vi "CVSUI.vi"() -> ()   [LabVIEW 2013, in "PLTarget CVS.lvclass"]
uses:
  PLTarget CVS.lvclass
  <vilib>/NI/Configuration Framework/Node/NodeRef.ctl
  <vilib>/NI/Configuration Framework/Node/NISE_CEF_Node.lvclass
  <vilib>/NI/AMC/Message Queue.ctl
  <vilib>/NI/AMC/Message.ctl
  <vilib>/NI/Tools/Keyed Array/KeyedArray.ctl
  <vilib>/NI/Configuration Framework/Node/UserEventRef.ctl
  <vilib>/NI/Configuration Framework/Controls/EventCluster.ctl
  <vilib>/NI/Tag Bus Module Framework/root configuration/Target Types.ctl
  <vilib>/NI/Configuration Framework/Node/RefreshUIEvent.ctl
  <vilib>/NI/Configuration Framework/Node/CacheState.ctl
  <vilib>/NI/Configuration Framework/Node/StopEvent.ctl
  <vilib>/NI/Configuration Framework/Node/NodeChangeEvent.ctl
  Configuration Editor/Classes/TBM Configuration Node/deployment configuration.ctl
  Configuration Editor/Classes/Targets/Targets.lvclass/Targets.ctl
  PLTarget CVS.lvclass/PLTarget CVS.ctl
  Framework Configuration Classes/target configuration/PL_Target Configuration.lvclass/PL_Target Configuration.ctl
  <vilib>/NI/Configuration Framework/serializable node/NISE_CEF_serializable node.lvclass
  <vilib>/NI/Tag Bus Module Framework/root configuration/TBM configuration.lvclass
  Configuration Editor/Classes/Targets/Write additional files.vi
  Configuration Editor/Classes/Targets/Read additional files.vi
  <vilib>/NI/Configuration Framework/serializable configuration/set alias.vi
  <vilib>/NI/Configuration Framework/serializable configuration/get alias.vi
  <vilib>/NI/Configuration Framework/serializable configuration/NISE_CEF_serializable configuration.lvclass
  Framework Configuration Classes/target configuration/PL_Target Configuration.lvclass
  Configuration Editor/Classes/Targets/Targets.lvclass
  <vilib>/NI/Tools/Keyed Array/Tools_KeyedArray.lvlib
  <vilib>/NI/AMC/AMC.lvlib
  <vilib>/NI/Configuration Framework/NISE_CEF_TreeControl.lvlib
  Configuration Editor/Classes/TBM Configuration Node/TBM Configuration Node.lvclass
panel:
  in  "additional files":T1[](array[typedef])
  in  "node change":T2
  in  "stop event":T3
  in  "cache state":T4
  in  "refresh UI":T5
  in  "open fp?":bool=TRUE
  in  "generate includes file":bool
  in  "Includes file path":path
  in  "Local Bitfile Path":path
  in  "load bitfile":bool
  in  "bitfile path on target relative to root (c:\\ or /home/lvuser/)":path
  in  "RIO FPGA":string="RIO0"
  in  "Target Type":T6=enum."Linux RT ARM"
  in  "path to deploy on target relative to root (c:\\ or /home/lvuser/)":path
  in  "IP":string
  in  "user event":T7
  in  "main queue":T8
  in  "Name":string
  in  "node ref":T9
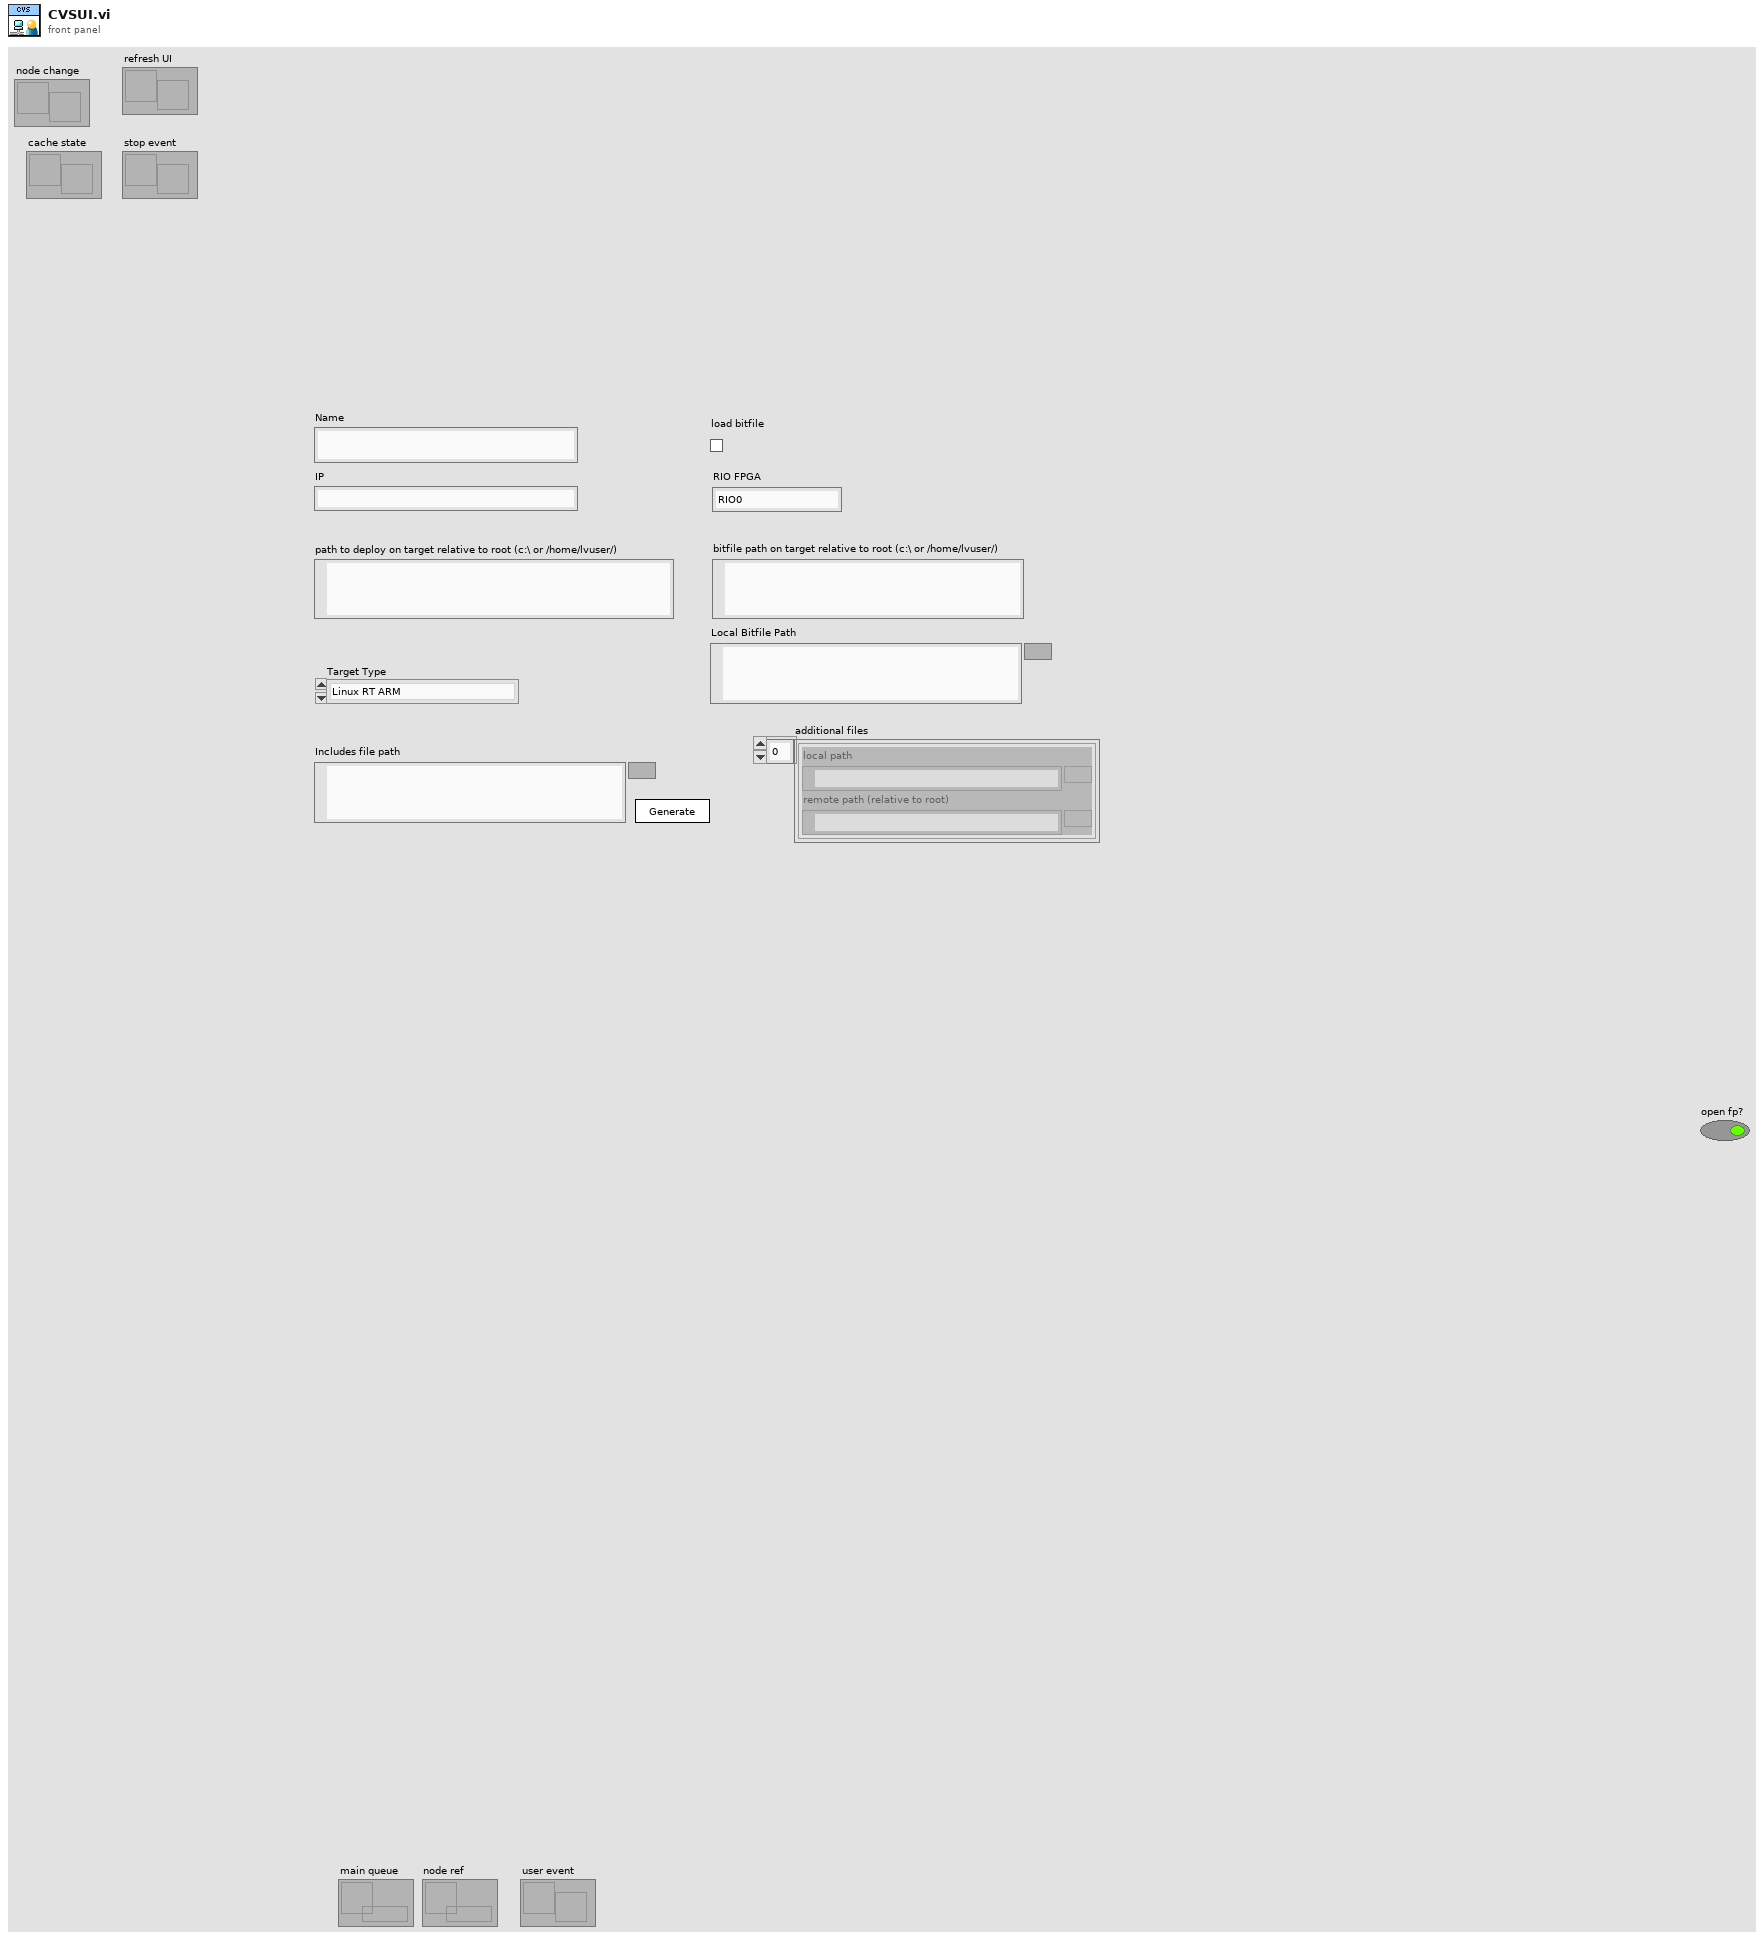
[diagram p1: front panel]
types:
  T1 = typedef "PL Framework Configuration Tool.lvlib/TBM Configuration Node.lvclass/deployment configuration.ctl" = cluster{"local path":path, "remote path (relative to root)":path}
  T2 = typedef "NISE_CEF_Node.lvclass/NodeChangeEvent.ctl" = refnum<user-event>
  T3 = typedef "NISE_CEF_Node.lvclass/StopEvent.ctl" = refnum<user-event>
  T4 = typedef "NISE_CEF_Node.lvclass/CacheState.ctl" = refnum<user-event>
  T5 = typedef "NISE_CEF_Node.lvclass/RefreshUIEvent.ctl" = refnum<user-event>
  T6 = typedef "TBM configuration.lvclass/Target Types.ctl" = enum16{"Windows", "Mac", "Linux", "Linux RT ARM", "VxWorks", "Pharlap", "Other", "Linux RT x64"}
  T7 = typedef "NISE_CEF_Node.lvclass/UserEventRef.ctl" = refnum<user-event>
  T8 = typedef "AMC.lvlib/Message Queue.ctl" = refnum<queue>
  T9 = typedef "NISE_CEF_Node.lvclass/NodeRef.ctl" = refnum<data-value>
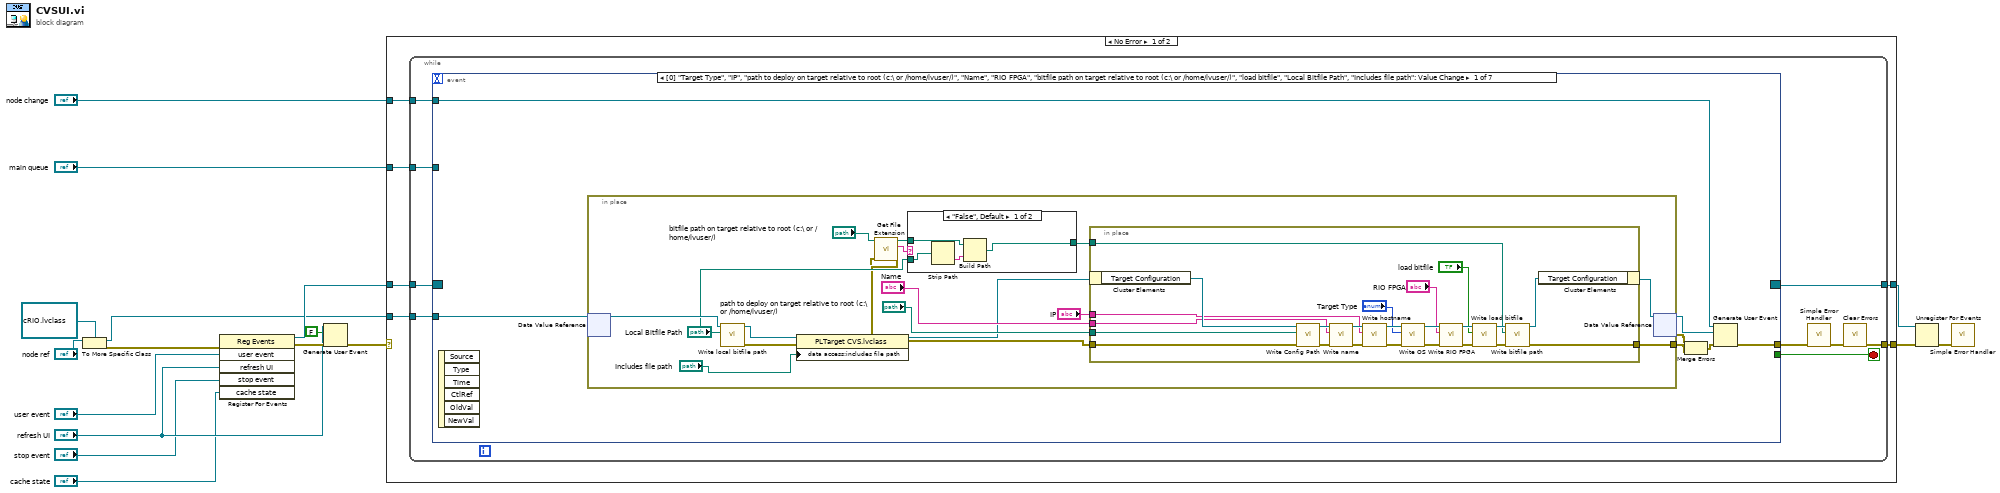
[diagram p0: block diagram]
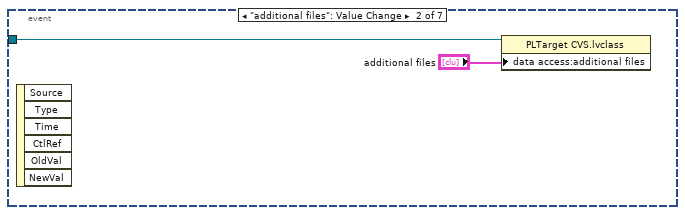
[diagram p3: hidden frame]
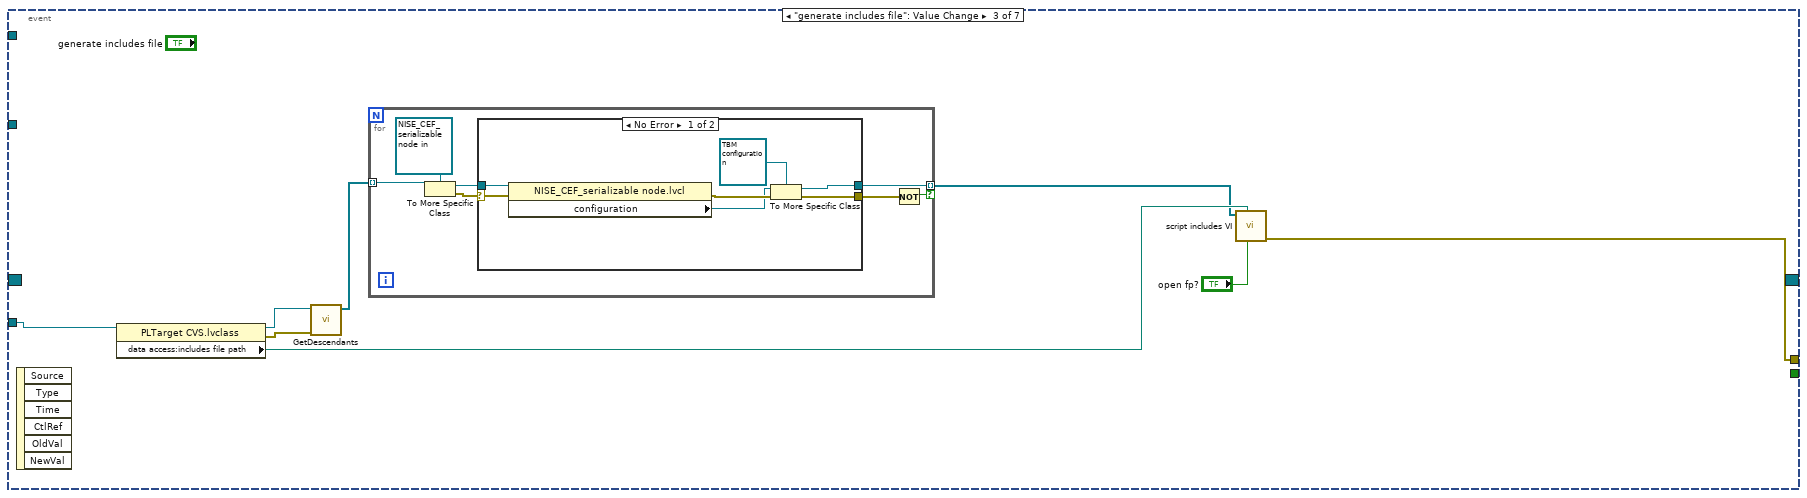
[diagram p4: hidden frame]
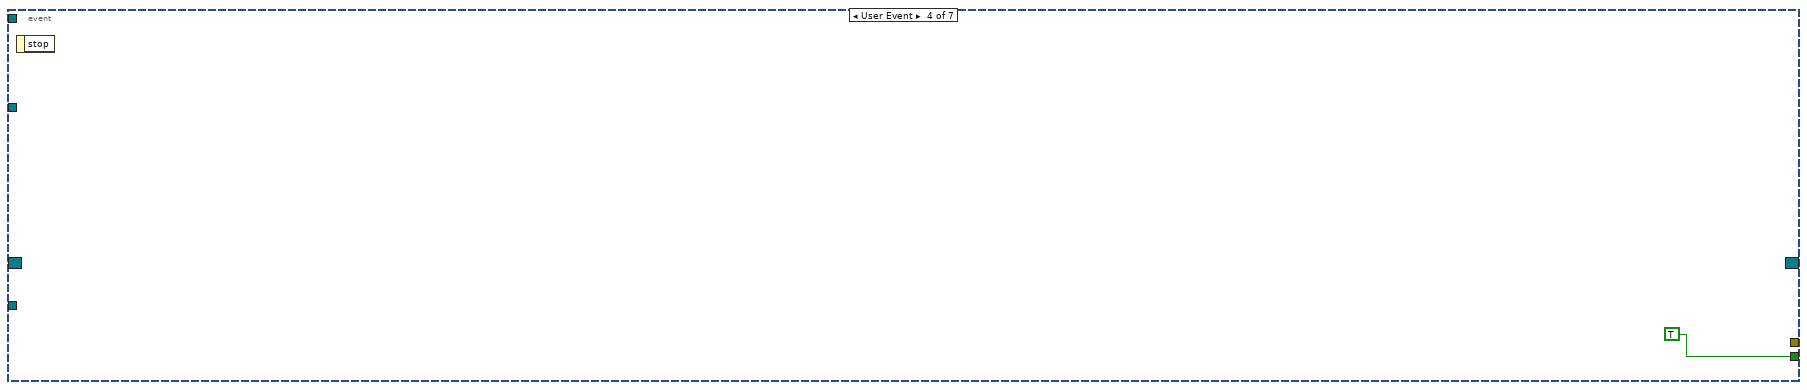
[diagram p6: hidden frame]
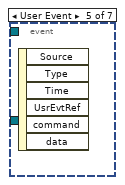
[diagram p7: hidden frame]
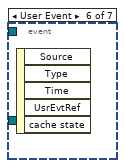
[diagram p8: hidden frame]
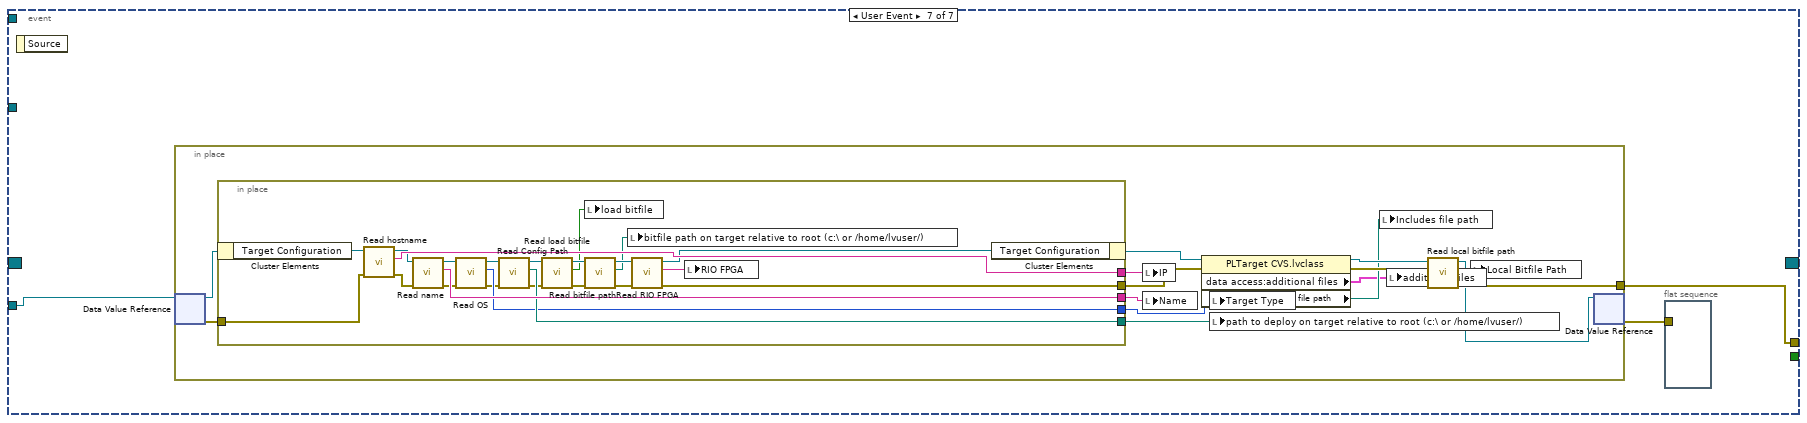
[diagram p9: hidden frame]
diagram:
  n1 = To More Specific Class(target class=refnum<data-value> refnum ("data value reference"), reference="node ref") -> (specific class reference=w4:refnum<data-value>, error out=w5:errorcluster)  [unwired: 1 in]
  n2 = register-events(error in=w5, "user event", "refresh UI", "stop event", "cache state") -> (reference out=w15:refnum<event-registration>, error out=w12:errorcluster)  [unwired: 1 in]
  n3 = Generate User Event(user event="refresh UI", event data cluster=FALSE ("event data"), error in=w12) -> (error out=w6:errorcluster)  [unwired: 1 in, 1 out]
  n4 = case shown="No Error" w6 {
    selector: w6 -> [_ w152]
    tunnel: w4 -> [w23 _]
    tunnel: "main queue" -> [w22 _]
    tunnel: w15 -> [w21 w153]
    tunnel: [w20 w153] -> w14
    tunnel: [w19 w152] -> w13
    tunnel: "node change" -> [w18 _]
    frame No Error {
      n5 = while {
        tunnel: w23 -> [w32]
        tunnel: w22 -> [w31]
        tunnel: w21 -> [w30]
        tunnel: [w29] -> w20
        tunnel: [w25] -> w19
        tunnel: w18 -> [w24]
        stop <- w28 stop-if-true
        n6 = event shown="[0] \"Target Type\", \"IP\", \"path to deploy on target relative to root (c:\\ or /home/lvuser/)\", \"Name\", \"RIO FPGA\", \"bitfile path on target relative to root (c:\\ or /home/lvuser/)\", \"load bitfile\", \"Local Bitfile Path\", \"Includes file path\": Value Change" {
          selector: w30 -> [_ _ _ _ _ _ _]
          dyn-events: [_ _ _ _ _ _ _] -> w29
          timeout: _ -> [_ _ _ _ _ _ _]
          tunnel: w32 -> [w39 w86 w94 _ _ _ w113]
          tunnel: w31 -> [_ _ _ _ _ _ _]
          tunnel: [_ _ _ TRUE _ _ _] -> w28
          tunnel: [w37 _ w91 _ _ _ w112] -> w27
          tunnel: w24 -> [w36 _ _ _ _ _ _]
          event "IP", "path to deploy on target relative to root (c:\\ or /home/lvuser/)", "Name", "RIO FPGA", "bitfile path on target relative to root (c:\\ or /home/lvuser/)", "load bitfile", "Local Bitfile Path", "Includes file path": Value Change {
            n7 = event-data() -> ()  [unwired: 1 in, 6 out]
            n8 = in-place {
              in-place-border: [w52] -> w38
              n9 = in-place-dvr #1(w39) -> (w51:refnum<class "PLTarget CVS.lvclass">)  [unwired: 1 out]
              n10 = call "Write local bitfile path.vi"("bitfile path"="Local Bitfile Path", "Targets in"=w51) -> ("error out"=w45:errorcluster, "Targets out"=w42:refnum<class "PLTarget CVS.lvclass">)  [unwired: 8 in]
              n11 = property class="PLTarget CVS.lvclass"(reference=w42, error in=w45, "data access:includes file path"="Includes file path") -> (reference out=w41:refnum<class "PLTarget CVS.lvclass">, error out=w43:errorcluster)
              n12 = call <vilib>:"Get File Extension.vi"("error in (no error)"=w43, "file"="bitfile path on target relative to root (c:\\ or /home/lvuser/)") -> ("error out"=w44:errorcluster, "lowercase file extension"=w49:string, "dup file"=w47:path)  [unwired: 6 in, 1 out]
              n13 = case shown="\"False\", Default" w49 {
                tunnel: [w59 w61] -> w48
                tunnel: w47 -> [w60 w61]
                tunnel: "Local Bitfile Path" -> [w57 _]
                frame "False", Default {
                  n14 = Strip Path(path=w57) -> (name=w58:string)  [unwired: 1 out]
                  n15 = Build Path(base path=w60, name or relative path=w58) -> (appended path=w59:path)
                }
                frame "lvbit", "lvbitx" {
                }
              }
              n16 = in-place {
                in-place-border: "path to deploy on target relative to root (c:\\ or /home/lvuser/)" -> [w83]
                in-place-border: "IP" -> [w80]
                in-place-border: "Name" -> [w79]
                in-place-border: w44 -> [w66]
                in-place-border: [w65] -> w52
                in-place-border: w48 -> [w62]
                n17 = in-place-cluster #2(w41) -> ("Target Configuration"=w84:refnum<class "PL_Target Configuration.lvclass">)
                n18 = call "Write Config Path.vi"("error in"=w66, "Config Path"=w83, "PL_Local Target Configuration in"=w84) -> ("error out"=w70:errorcluster, "PL_Local Target Configuration out"=w82:refnum<class "PL_Target Configuration.lvclass">)  [unwired: 7 in]
                n19 = call "Write name.vi"("error in"=w70, "name"=w79, "PL_Local Target Configuration in"=w82) -> ("error out"=w69:errorcluster, "PL_Local Target Configuration out"=w81:refnum<class "PL_Target Configuration.lvclass">)  [unwired: 7 in]
                n20 = call "Write hostname.vi"("error in"=w69, "hostname"=w80, "PL_Target Configuration in"=w81) -> ("error out"=w68:errorcluster, "PL_Target Configuration out"=w78:refnum<class "PL_Target Configuration.lvclass">)  [unwired: 7 in]
                n21 = call "Write OS.vi"("error in"=w68, "Target Types"="Target Type", "PL_Target Configuration in"=w78) -> ("error out"=w67:errorcluster, "PL_Target Configuration out"=w72:refnum<class "PL_Target Configuration.lvclass">)  [unwired: 7 in]
                n22 = call "Write RIO FPGA.vi"("error in"=w67, "RIO FPGA"="RIO FPGA", "PL_Target Configuration in"=w72) -> ("error out"=w74:errorcluster, "PL_Target Configuration out"=w73:refnum<class "PL_Target Configuration.lvclass">)  [unwired: 7 in]
                n23 = call "Write load bitfile.vi"("error in"=w74, "load bitfile"="load bitfile", "PL_Target Configuration in"=w73) -> ("error out"=w76:errorcluster, "PL_Target Configuration out"=w75:refnum<class "PL_Target Configuration.lvclass">)  [unwired: 7 in]
                n24 = call "Write bitfile path.vi"("error in"=w76, "bitfile path"=w62, "PL_Target Configuration in"=w75) -> ("error out"=w65:errorcluster, "PL_Target Configuration out"=w71:refnum<class "PL_Target Configuration.lvclass">)  [unwired: 7 in]
                n25 = in-place-cluster #2("Target Configuration"=w71) -> (w56:refnum<class "PLTarget CVS.lvclass">)
              }
              n26 = in-place-dvr #1(w56) -> (w35:refnum<data-value>, w33:errorcluster)
            }
            n27 = Merge Errors(w38, w33) -> (w34:errorcluster)
            n28 = Generate User Event(user event=w36, event data cluster=w35, error in=w34) -> (error out=w37:errorcluster)  [unwired: 1 in, 1 out]
          }
          event "additional files": Value Change {
            n29 = event-data() -> ()  [unwired: 1 in, 6 out]
            n30 = property class="PLTarget CVS.lvclass"(reference=w86, "data access:additional files"="additional files") -> ()  [unwired: 1 in, 2 out]
          }
          event "generate includes file": Value Change {
            n31 = event-data() -> ()  [unwired: 1 in, 6 out]
            n32 = property class="PLTarget CVS.lvclass"(reference=w94) -> (reference out=w89:refnum<data-value>, error out=w90:errorcluster, "data access:includes file path"=w92:path)  [unwired: 1 in]
            n33 = call <vilib>:"GetDescendants.vi"("error in"=w90, "node in"=w89) -> ("descendants"=w88:refnum<data-value>[])  [unwired: 8 in, 1 out]
            n34 = for {
              tunnel: w88 -> [w101] mode=indexing
              tunnel: [w97] -> w87 mode=indexing if=w95
              n35 = To More Specific Class(target class=refnum<data-value> refnum, reference=w101) -> (specific class reference=w98:refnum<data-value>, error out=w99:errorcluster)  [unwired: 1 in]
              n36 = case shown="No Error" w99 {
                selector: w99 -> [w107 w109]
                tunnel: w98 -> [w108 _]
                tunnel: [w102 _] -> w97
                tunnel: [w105 w109] -> w96
                frame No Error {
                  n37 = property class="NISE_CEF_serializable node.lvcl"(reference=w108, error in=w107) -> (error out=w106:errorcluster, "configuration"=w104:refnum<class "NISE_CEF_serializable configuration.lvclass">)  [unwired: 1 out]
                  n38 = To More Specific Class(target class=refnum<class "TBM configuration.lvclass"> refnum ("configuration"), reference=w104, error in=w106) -> (specific class reference=w102:refnum<class "TBM configuration.lvclass">, error out=w105:errorcluster)
                }
                frame Error {
                }
              }
              n39 = Not(x=w96) -> (.not. x?=w95:bool)
            }
            n40 = call "script includes VI.vi"("open fp?"="open fp?", "vi path (blank=new)"=w92, "cfg objects"=w87) -> ("error out"=w91:errorcluster)  [unwired: 8 in]
          }
          event User Event {
            n41 = event-data() -> ()  [unwired: 1 in, 1 out]
          }
          event User Event {
            n42 = event-data() -> ()  [unwired: 1 in, 6 out]
          }
          event User Event {
            n43 = event-data() -> ()  [unwired: 1 in, 5 out]
          }
          event User Event {
            n44 = event-data() -> ()  [unwired: 1 in, 1 out]
            n45 = in-place {
              in-place-border: [w121] -> w112
              n46 = in-place-dvr #3(w113) -> (w125:refnum<class "PLTarget CVS.lvclass">, w123:errorcluster)
              n47 = in-place {
                in-place-border: [w151] -> w128
                in-place-border: [w146] -> w126
                in-place-border: [w150] -> w127
                in-place-border: [w144] -> w124
                in-place-border: w123 -> [w133]
                in-place-border: [w132] -> w122
                n48 = in-place-cluster #4(w125) -> ("Target Configuration"=w147:refnum<class "PL_Target Configuration.lvclass">)
                n49 = call "Read hostname.vi"("error in"=w133, "PL_Target Configuration in"=w147) -> ("error out"=w143:errorcluster, "hostname"=w150:string, "PL_Target Configuration out"=w148:refnum<class "PL_Target Configuration.lvclass">)  [unwired: 7 in]
                n50 = call "Read name.vi"("error in"=w143, "PL_Local Target Configuration in"=w148) -> ("error out"=w142:errorcluster, "name"=w151:string, "PL_Local Target Configuration out"=w149:refnum<class "PL_Target Configuration.lvclass">)  [unwired: 7 in]
                n51 = call "Read OS.vi"("error in"=w142, "PL_Target Configuration in"=w149) -> ("error out"=w141:errorcluster, "Target Types"=w144:T6, "PL_Target Configuration out"=w145:refnum<class "PL_Target Configuration.lvclass">)  [unwired: 7 in]
                n52 = call "Read Config Path.vi"("error in"=w141, "PL_Local Target Configuration in"=w145) -> ("error out"=w134:errorcluster, "Config Path"=w146:path, "PL_Local Target Configuration out"=w135:refnum<class "PL_Target Configuration.lvclass">)  [unwired: 7 in]
                n53 = call "Read load bitfile.vi"("error in"=w134, "PL_Target Configuration in"=w135) -> ("error out"=w138:errorcluster, "load bitfile"=w129:bool, "PL_Target Configuration out"=w137:refnum<class "PL_Target Configuration.lvclass">)  [unwired: 7 in]
                n54 = local write "load bitfile"(w129) -> ()
                n55 = call "Read bitfile path.vi"("error in"=w138, "PL_Target Configuration in"=w137) -> ("error out"=w140:errorcluster, "bitfile path"=w130:path, "PL_Target Configuration out"=w139:refnum<class "PL_Target Configuration.lvclass">)  [unwired: 7 in]
                n56 = local write "bitfile path on target relative to root (c:\\ or /home/lvuser/)"(w130) -> ()
                n57 = call "Read RIO FPGA.vi"("error in"=w140, "PL_Target Configuration in"=w139) -> ("error out"=w132:errorcluster, "RIO FPGA"=w131:string, "PL_Target Configuration out"=w136:refnum<class "PL_Target Configuration.lvclass">)  [unwired: 7 in]
                n58 = local write "RIO FPGA"(w131) -> ()
                n59 = in-place-cluster #4("Target Configuration"=w136) -> (w117:refnum<class "PLTarget CVS.lvclass">)
              }
              n60 = local write "IP"(w127) -> ()
              n61 = local write "Name"(w128) -> ()
              n62 = property class="PLTarget CVS.lvclass"(reference=w117, error in=w122) -> (reference out=w116:refnum<class "PLTarget CVS.lvclass">, error out=w118:errorcluster, "data access:additional files"=w114:T1[], "data access:includes file path"=w115:path)
              n63 = local write "Target Type"(w124) -> ()
              n64 = local write "path to deploy on target relative to root (c:\\ or /home/lvuser/)"(w126) -> ()
              n65 = local write "Includes file path"(w115) -> ()
              n66 = local write "additional files"(w114) -> ()
              n67 = call "Read local bitfile path.vi"("error in"=w118, "Targets in"=w116) -> ("error out"=w121:errorcluster, "bitfile path"=w119:path, "Targets out"=w120:refnum<class "PLTarget CVS.lvclass">)  [unwired: 7 in]
              n68 = local write "Local Bitfile Path"(w119) -> ()
              n69 = in-place-dvr #3(w120) -> (w111:errorcluster)  [unwired: 1 out]
            }
            n70 = flat-sequence {
              tunnel: w111 -> [_]
              frame #0 {
              }
            }
          }
        }
        n71 = call <vilib>:"Simple Error Handler.vi"("error in (no error)"=w27) -> ("error out"=w26:errorcluster)  [unwired: 4 in, 4 out]
        n72 = call <vilib>:"Clear Errors.vi"("error in (no error)"=w26) -> ("error out"=w25:errorcluster)  [unwired: 6 in]
      }
    }
    frame Error {
    }
  }
  n73 = Unregister For Events(event registration refnum=w14, error in=w13) -> (error out=w3:errorcluster)
  n74 = call <vilib>:"Simple Error Handler.vi"("error in (no error)"=w3) -> ()  [unwired: 4 in, 5 out]
